vi "Tell If Stopped.vi"(4 "Priority":bool, 9 "Msg":refnum<class "Msg.lvclass">, 10 "Transport":refnum<class "Transport.lvclass">) -> (0 "Error out":errorcluster)   [LabVIEW 2025, in "jettl.lvlib"]
uses:
  jettl.lvlib
  Msg/Msg.lvclass
  Transport/Transport.lvclass
  Stopped jettl Msg/Stopped/Init Msg Default.vi
  Stopped jettl Msg/Stopped/Stopped.lvlib
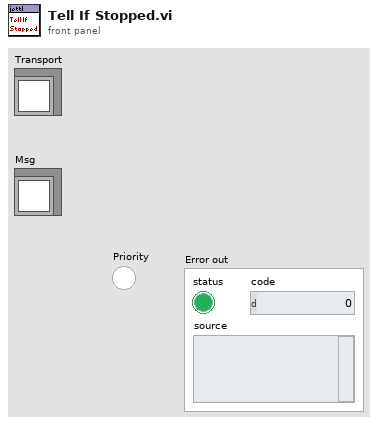
[diagram p1: front panel]
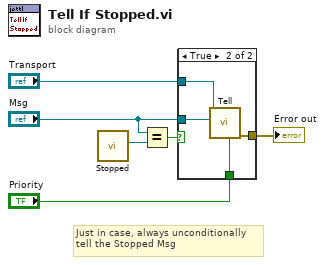
[diagram p0: block diagram]
diagram:
  # "Just in case, always unconditionally tell the Stopped Msg"
  n1 = call-poly "Stopped.vi"() -> ("Msg"=w6:refnum<class "Msg.lvclass">)  [unwired: 11 in]
  n2 = Equal?(x="Msg", y=w6) -> (x = y?=w5:bool)
  n3 = case shown="True" w5 {
    tunnel: "Transport" -> [_ w10]
    tunnel: "Priority" -> [_ w9]
    tunnel: [_ w8] -> w4
    tunnel: "Msg" -> [_ w7]
    frame False {
    }
    frame True {
      n4 = call-dynamic "Tell.vi"("Priority"=w9, "Msg"=w7, "Transport in"=w10) -> ("Error out"=w8:errorcluster)  [unwired: 8 in]
    }
  }
  "Error out" <- w4
